vi "T1_meas_freq.vi"() -> ()   [LabVIEW 2014]
uses:
  <vilib>/Utility/file.llb/Write To Spreadsheet File (DBL).vi
  <vilib>/Utility/file.llb/Read From Spreadsheet File (DBL).vi
  <vilib>/gmath/NumericalOptimization/Nonlinear Curve Fit LM formula string.vi
  <vilib>/gmath/NI_Gmath.lvlib
  <vilib>/Analysis/NI_AALBase.lvlib
panel:
  in  "semester":string(combo)="ws17"
  out "subarray":dbl[](array[numeric])=[20.0, 40.0, 60.0, 100.0, 140.0, 180.0, 300.0, 360.0, 600.0, 800.0]
  out "appended array":dbl[](array[numeric])=[1000.0, -2000.0, 100.0]
  in  "Y-range low":dbl
  out "A":dbl[](array[numeric]) format="%.1f"
  out "T1[ms]":dbl[](array[numeric]) format="%.1f"
  out "error T1[ms]":dbl[](array[numeric]) format="%.1f"
  out "error A":dbl[](array[numeric]) format="%.1f"
  out "T1_i[ms]":dbl=100.0
  out "A_i":dbl=1000.0
  in  "Y-range high":dbl=200.0
  in  "X-range":dbl=1500.0
  out "hlim":dbl=1197.4683544303798 format="%#.1f"
  out "llim":dbl=824.4725738396625 format="%#.1f"
  out "spin echo\nsignal":dbl=7.876213904626598
  in  "time-out":u32=6
  in  "gain":u32=1000
  out "Fourier spectrum":cluster{"Y":dbl[], "Y":dbl[]}[](graph)
  in  "del T (+-)":u32=10
  in  "folder":string
  in  "don`t write data, update plot, no fit:":bool
  in  "fit:":bool
  out "XY Graph":cluster{"Y":dbl[], "Y":dbl[]}[](graph) caption="Data"
  out "error echo amplv":dbl[](array[numeric])=[0.074] format="%.3f"
  out "echo amplv":dbl[](array[numeric])=[0.745] format="%.2f"
  out "echo timev":dbl[](array[numeric])=[100.0] format="%#.1f"
  in  "many measurements:":bool=TRUE
  out "x+y":i32=2
  in  "data file":string
  out "error avg peak":dbl format="%.3f"
  out "avg peak":dbl format="%.2f"
  out "amplitude window":cluster{"Y":dbl[], "Y":dbl[]}[](graph)
  out "amplitude":cluster{"Y":dbl[], "Y":dbl[]}[](graph) caption="XY Graph"
  in  "scan freq [kHz]":u32=10
  in  "meas. time":u32=200
  in  "number meas":i32=10
  in  "spin echo time":u32=80
  in  "write data to file, update plot:":bool
  in  "single measurement:":bool=TRUE
  in  "stop":bool=TRUE
  # "peak window"
  # "1)"
  # "2)"
  # "data measured:"
  # "3)"
  # "4)"
  # "5)"
  # "fit values:"
  # "init values:"
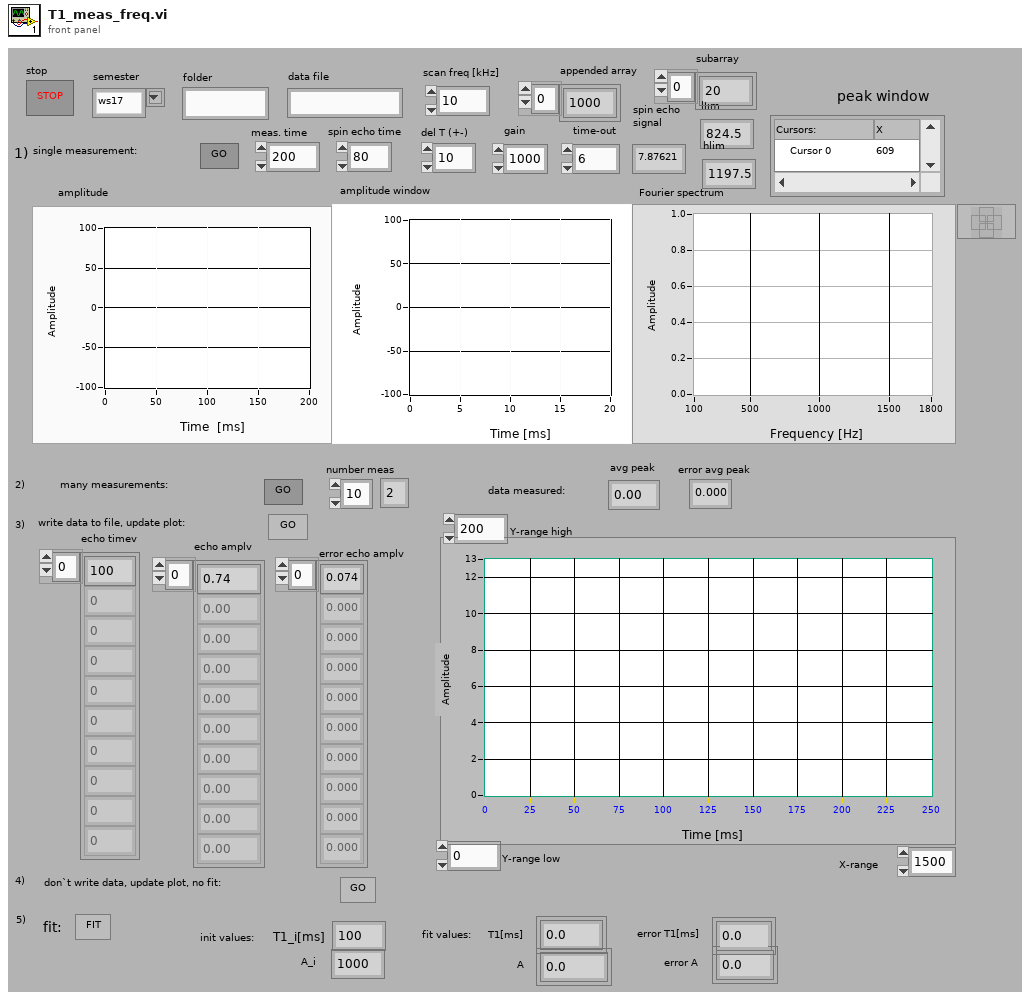
[diagram p1: front panel]
types:
  T1 = cluster{"model":string, "Parameters":string[], "x":string}
  T2 = typedef "LVCursorListTypeDef.ctl" = cluster{"Name":string, "Color":u32, "Style":u8, "Point Style":u8, "Name Visible":bool, "Allow Drag":bool, "Cursor Mode":u32, "Plot":i32, "Index":i32, "Position":cluster{"X":dbl, "Y":dbl}, "X Scale":u32, "Y Scale":u32, "Watch Plots":i32[], "Watch All Plots":bool, "Plot Area":i32, "Label Offset":cluster{"X":dbl, "Y":dbl}}[]
  T3 = typedef "NI_Matrix.lvlib/RealMatrix.ctl" = dbl[][]
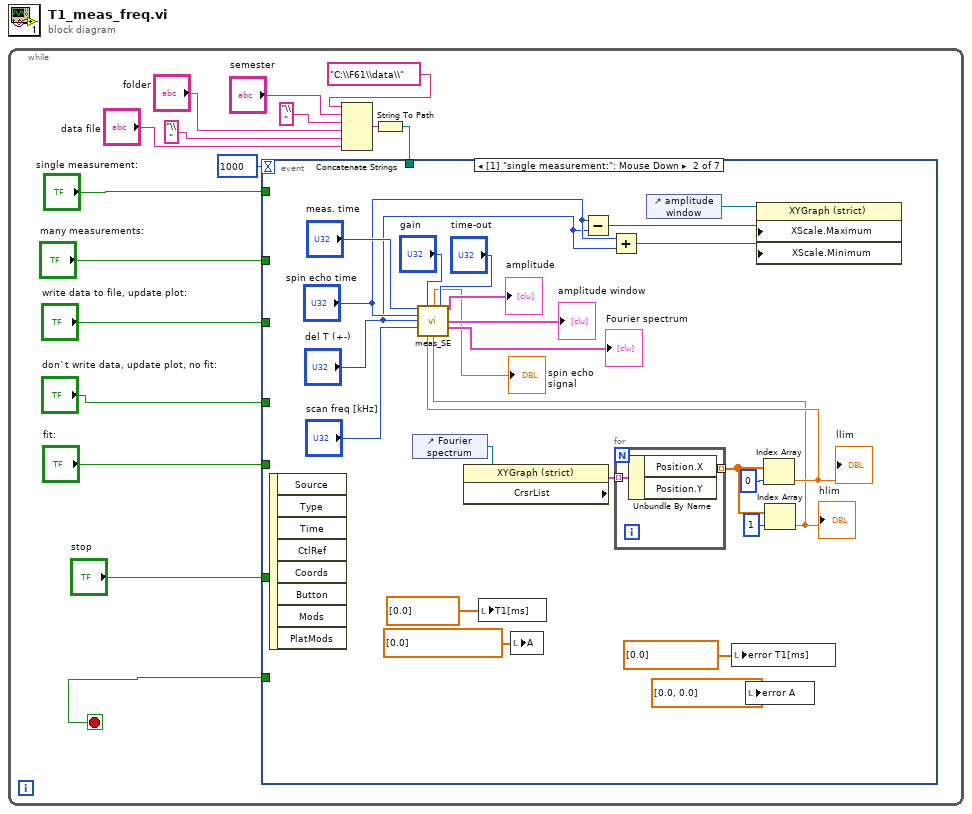
[diagram p0: block diagram]
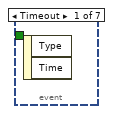
[diagram p2: hidden frame]
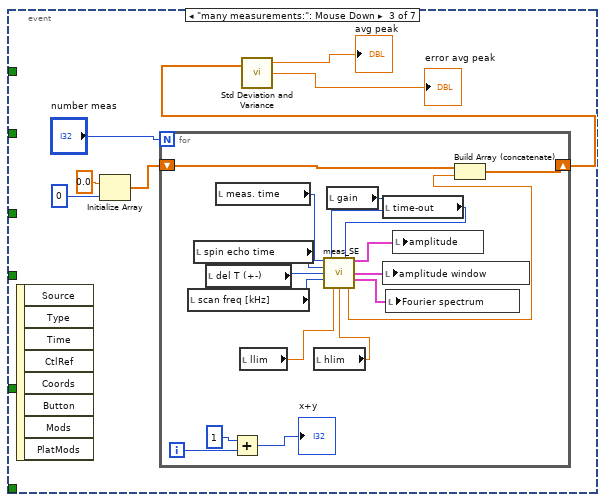
[diagram p3: hidden frame]
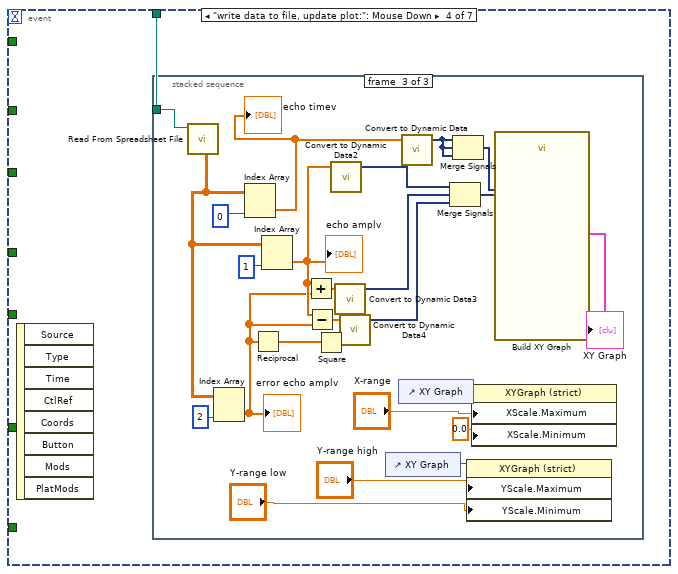
[diagram p4: hidden frame]
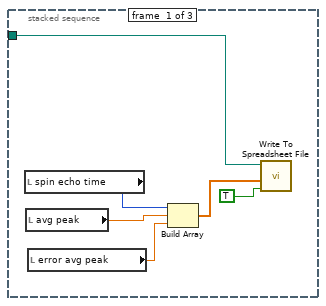
[diagram p5: hidden frame]
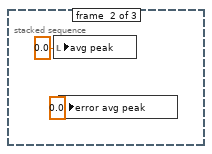
[diagram p6: hidden frame]
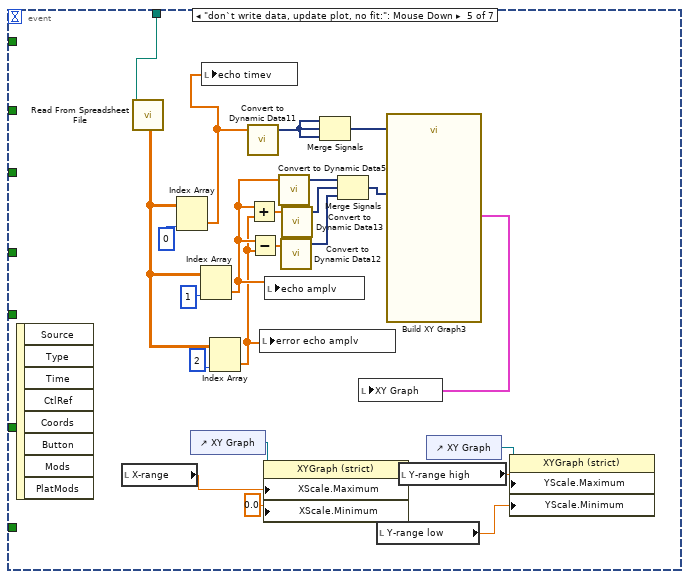
[diagram p7: hidden frame]
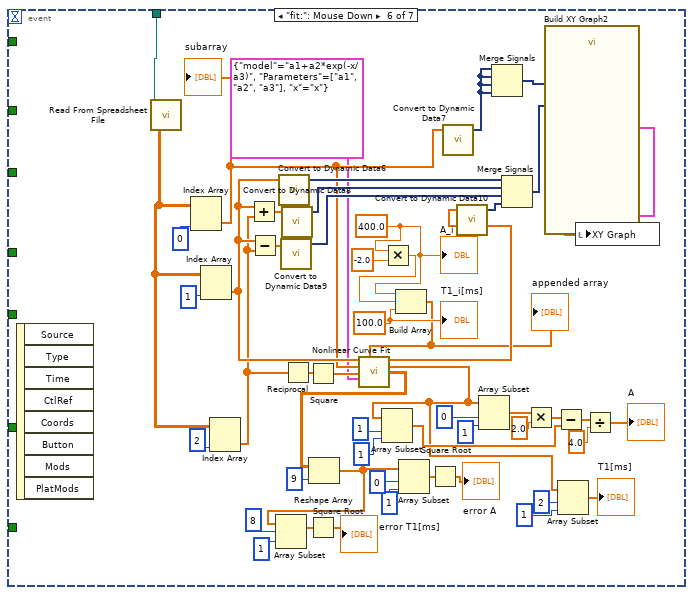
[diagram p8: hidden frame]
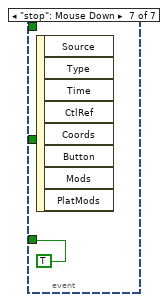
[diagram p9: hidden frame]
diagram:
  n1 = while {
    stop <- w9 stop-if-true
    n2 = Concatenate Strings("C:\\F61\\data\\", "semester", "\\" ("string"), "folder", "\\" ("string"), "data file") -> (w14:string)
    n3 = String To Path(string=w14) -> (path=w13:path)
    n4 = event shown="[1] \"single measurement:\": Mouse Down" {
      selector: _ -> [_ _ _ _ _ _ _]
      dyn-events: _ -> [_ _ _ _ _ _ _]
      timeout: 1000 -> [_ _ _ _ _ _ _]
      tunnel: "single measurement:" -> [_ _ _ _ _ _ _]
      tunnel: "write data to file, update plot:" -> [_ _ _ _ _ _ _]
      tunnel: w13 -> [_ _ _ w67 w111 w157 _]
      tunnel: "many measurements:" -> [_ _ _ _ _ _ _]
      tunnel: "fit:" -> [_ _ _ _ _ _ _]
      tunnel: "stop" -> [_ _ _ _ _ _ _]
      tunnel: [_ _ _ _ _ _ TRUE ("stop")] -> w9
      tunnel: "don`t write data, update plot, no fit:" -> [_ _ _ _ _ _ _]
      event Timeout {
        n5 = event-data() -> ()  [unwired: 1 in, 2 out]
      }
      event "single measurement:": Mouse Down {
        n6 = event-data() -> ()  [unwired: 1 in, 8 out]
        n7 = control-ref of="Fourier spectrum"() -> (w40:refnum<vi>)
        n8 = property class="XYGraph (strict)"(reference=w40) -> ("CrsrList"=w39:T2)  [unwired: 1 in, 2 out]
        n9 = local write "T1[ms]"(dbl[] [0.0] ("T1[ms]")) -> ()
        n10 = local write "A"(dbl[] [0.0] ("A")) -> ()
        n11 = Subtract(x="spin echo time", y="del T (+-)") -> (x-y=w23:u32)
        n12 = Add(x="spin echo time", y="del T (+-)") -> (x+y=w22:u32)
        n13 = for {
          tunnel: w39 -> [w42] mode=indexing
          tunnel: [w41] -> w38 mode=indexing
          n14 = Unbundle By Name(w42) -> ("Position.X"=w41:dbl)  [unwired: 1 out]
        }
        n15 = control-ref of="amplitude window"() -> (w26:refnum<vi>)
        n16 = local write "error T1[ms]"(dbl[] [0.0] ("error T1[ms]")) -> ()
        n17 = local write "error A"(dbl[] [0.0, 0.0] ("error A")) -> ()
        n18 = property class="XYGraph (strict)"(reference=w26, "XScale.Maximum"=w23, "XScale.Minimum"=w22) -> ()  [unwired: 1 in, 2 out]
        n19 = Index Array(array=w38, index=0) -> (element=w28:dbl)
        "llim" <- w28
        n20 = Index Array(array=w38, index=1) -> (element=w27:dbl)
        "hlim" <- w27
        n21 = call "meas_SE.vi"("meas. time [ms]"="meas. time", "gainfac"="gain", "time out [s]"="time-out", "spin echo time [ms]"="spin echo time", "del T (+-) ][ms]"="del T (+-)", "scan freq [kHz]"="scan freq [kHz]", "llim"=w28, "hlim"=w27) -> ("SE"=→"spin echo\nsignal":dbl, "Amplitude"=→"amplitude":cluster{"Y":dbl[], "Y":dbl[]}[], "Spin echo (time)"=→"amplitude window":cluster{"Y":dbl[], "Y":dbl[]}[], "Spin echo (freq)"=→"Fourier spectrum":cluster{"Y":dbl[], "Y":dbl[]}[])  [unwired: 3 in, 1 out]
      }
      event "many measurements:": Mouse Down {
        n22 = event-data() -> ()  [unwired: 1 in, 8 out]
        n23 = Initialize Array(0.0 ("element"), 0 ("dimension size")) -> (w47:dbl[])
        n24 = for {
          N: "number meas" -> [_]
          shift-right: [w62] -> w46
          shift-left: w47 -> [w63]
          i -> [w65]
          n25 = local read "scan freq [kHz]"() -> (w58:u32)
          n26 = local read "spin echo time"() -> (w60:u32)
          n27 = local read "del T (+-)"() -> (w59:u32)
          n28 = local read "meas. time"() -> (w61:u32)
          n29 = Add(x=1, y=w65) -> (x+y=→"x+y":i32)
          n30 = local read "llim"() -> (w54:dbl)
          n31 = local read "hlim"() -> (w53:dbl)
          n32 = local read "gain"() -> (w57:u32)
          n33 = local read "time-out"() -> (w56:u32)
          n34 = call "meas_SE.vi"("meas. time [ms]"=w61, "gainfac"=w57, "time out [s]"=w56, "spin echo time [ms]"=w60, "del T (+-) ][ms]"=w59, "scan freq [kHz]"=w58, "llim"=w54, "hlim"=w53) -> ("Amplitude"=w52:cluster{"Y":dbl[], "Y":dbl[]}[], "Spin echo (time)"=w51:cluster{"Y":dbl[], "Y":dbl[]}[], "Spin echo (freq)"=w50:cluster{"Y":dbl[], "Y":dbl[]}[], "SE-corr"=w55:dbl)  [unwired: 3 in, 1 out]
          n35 = local write "amplitude window"(w51) -> ()
          n36 = local write "Fourier spectrum"(w50) -> ()
          n37 = local write "amplitude"(w52) -> ()
          n38 = Build Array (concatenate)(w63, w55) -> (w62:dbl[])
        }
        n39 = call <vilib>:"Std Deviation and Variance.vi"("X"=w46) -> ("mean"=→"avg peak":dbl, "standard deviation"=→"error avg peak":dbl)  [unwired: 1 in, 1 out]
      }
      event "write data to file, update plot:": Mouse Down {
        n40 = event-data() -> ()  [unwired: 1 in, 8 out]
        n41 = stacked-sequence {
          tunnel: w67 -> [w68 _ w99]
          frame #0 {
            n42 = local read "spin echo time"() -> (w69:u32)
            n43 = local read "avg peak"() -> (w70:dbl)
            n44 = local read "error avg peak"() -> (w73:dbl)
            n45 = Build Array(w69, w70, w73) -> (w71:dbl[])
            n46 = call-poly <vilib>:"Write To Spreadsheet File.vi"("append to file? (new file:F)"=TRUE, "1D data"=w71, "file path (dialog if empty)"=w68) -> ()  [unwired: 5 in, 1 out]
          }
          frame #1 {
            n47 = local write "avg peak"(sgl 0.0 ("avg diff")) -> ()
            n48 = local write "error avg peak"(0.0 ("error avg diff")) -> ()
          }
          frame #2 {
            n49 = call-poly <vilib>:"Read From Spreadsheet File.vi"("file path (dialog if empty)"=w99) -> ("all rows"=w98:dbl[][])  [unwired: 6 in, 4 out]
            n50 = Index Array(array=w98, index (col)=2 ("index (row)")) -> (element=w84:dbl[])  [unwired: 1 in]
            "error echo amplv" <- w84
            n51 = Index Array(array=w98, index (col)=0 ("index (row)")) -> (element=w82:dbl[])  [unwired: 1 in]
            "echo timev" <- w82
            n52 = Reciprocal(x=w84) -> (1/x=w83:dbl[])
            n53 = Index Array(array=w98, index (col)=1 ("index (row)")) -> (element=w85:dbl[])  [unwired: 1 in]
            "echo amplv" <- w85
            n54 = Add(x=w85, y=w84) -> (x+y=w89:dbl[])
            n55 = Subtract(x=w85, y=w84) -> (x-y=w88:dbl[])
            n56 = Square(x=w83) -> ()  [unwired: 1 out]
            n57 = call "Convert to Dynamic Data2"("Array"=w85) -> ("Dynamic Data Type"=w90:dynamicdata)  [unwired: 3 in]
            n58 = call "Convert to Dynamic Data3"("Array"=w89) -> ("Dynamic Data Type"=w87:dynamicdata)  [unwired: 3 in]
            n59 = call "Convert to Dynamic Data4"("Array"=w88) -> ("Dynamic Data Type"=w86:dynamicdata)  [unwired: 3 in]
            n60 = control-ref of="XY Graph"() -> (w78:refnum<vi>)
            n61 = control-ref of="XY Graph"() -> (w81:refnum<vi>)
            n62 = call "Convert to Dynamic Data"("Array"=w82) -> ("Dynamic Data Type"=w93:dynamicdata)  [unwired: 3 in]
            n63 = Merge Signals(w90, w87, w86) -> (w91:dynamicdata)
            n64 = Merge Signals(w93, w93, w93) -> (w92:dynamicdata)
            n65 = property class="XYGraph (strict)"(reference=w78, "YScale.Maximum"="Y-range high", "YScale.Minimum"="Y-range low") -> ()  [unwired: 1 in, 2 out]
            n66 = property class="XYGraph (strict)"(reference=w81, "XScale.Maximum"="X-range", "XScale.Minimum"=0.0 ("X Scale.Range:Maximum")) -> ()  [unwired: 1 in, 2 out]
            n67 = call "Build XY Graph"("Y Input"=w91, "X Input"=w92) -> ("XY Graph"=→"XY Graph":cluster{"Y":dbl[], "Y":dbl[]}[])  [unwired: 8 in, 1 out]
          }
        }
      }
      event "don`t write data, update plot, no fit:": Mouse Down {
        n68 = event-data() -> ()  [unwired: 1 in, 8 out]
        n69 = local read "X-range"() -> (w104:dbl)
        n70 = call-poly <vilib>:"Read From Spreadsheet File.vi"("file path (dialog if empty)"=w111) -> ("all rows"=w122:dbl[][])  [unwired: 6 in, 4 out]
        n71 = Index Array(array=w122, index (col)=0 ("index (row)")) -> (element=w108:dbl[])  [unwired: 1 in]
        n72 = control-ref of="XY Graph"() -> (w103:refnum<vi>)
        n73 = Index Array(array=w122, index (col)=1 ("index (row)")) -> (element=w107:dbl[])  [unwired: 1 in]
        n74 = local write "echo timev"(w108) -> ()
        n75 = Index Array(array=w122, index (col)=2 ("index (row)")) -> (element=w106:dbl[])  [unwired: 1 in]
        n76 = call "Convert to Dynamic Data11"("Array"=w108) -> ("Dynamic Data Type"=w109:dynamicdata)  [unwired: 3 in]
        n77 = Add(x=w107, y=w106) -> (x+y=w115:dbl[])
        n78 = Subtract(x=w107, y=w106) -> (x-y=w114:dbl[])
        n79 = local write "error echo amplv"(w106) -> ()
        n80 = property class="XYGraph (strict)"(reference=w103, "XScale.Maximum"=w104, "XScale.Minimum"=0.0 ("X Scale.Range:Maximum")) -> ()  [unwired: 1 in, 2 out]
        n81 = local write "echo amplv"(w107) -> ()
        n82 = call "Convert to Dynamic Data5"("Array"=w107) -> ("Dynamic Data Type"=w116:dynamicdata)  [unwired: 3 in]
        n83 = call "Convert to Dynamic Data12"("Array"=w114) -> ("Dynamic Data Type"=w112:dynamicdata)  [unwired: 3 in]
        n84 = call "Convert to Dynamic Data13"("Array"=w115) -> ("Dynamic Data Type"=w113:dynamicdata)  [unwired: 3 in]
        n85 = Merge Signals(w109, w109, w109) -> (w118:dynamicdata)
        n86 = Merge Signals(w116, w113, w112) -> (w117:dynamicdata)
        n87 = local read "Y-range low"() -> (w100:dbl)
        n88 = call "Build XY Graph3"("Y Input"=w117, "X Input"=w118) -> ("XY Graph"=w110:cluster{"Y":dbl[], "Y":dbl[]}[])  [unwired: 8 in, 1 out]
        n89 = local write "XY Graph"(w110) -> ()
        n90 = local read "Y-range high"() -> (w101:dbl)
        n91 = control-ref of="XY Graph"() -> (w102:refnum<vi>)
        n92 = property class="XYGraph (strict)"(reference=w102, "YScale.Maximum"=w101, "YScale.Minimum"=w100) -> ()  [unwired: 1 in, 2 out]
      }
      event "fit:": Mouse Down {
        w150 = 100.0 ("element")
        w152 = 400.0 ("A")
        n93 = event-data() -> ()  [unwired: 1 in, 8 out]
        n94 = call-poly <vilib>:"Read From Spreadsheet File.vi"("file path (dialog if empty)"=w157) -> ("all rows"=w175:dbl[][])  [unwired: 6 in, 4 out]
        n95 = Index Array(array=w175, index (col)=0 ("index (row)")) -> (element=w158:dbl[])  [unwired: 1 in]
        "subarray" <- w158
        n96 = Index Array(array=w175, index (col)=1 ("index (row)")) -> (element=w164:dbl[])  [unwired: 1 in]
        n97 = Index Array(array=w175, index (col)=2 ("index (row)")) -> (element=w163:dbl[])  [unwired: 1 in]
        n98 = Add(x=w164, y=w163) -> (x+y=w168:dbl[])
        n99 = Subtract(x=w164, y=w163) -> (x-y=w167:dbl[])
        n100 = call "Convert to Dynamic Data6"("Array"=w164) -> ("Dynamic Data Type"=w169:dynamicdata)  [unwired: 3 in]
        n101 = call "Convert to Dynamic Data9"("Array"=w167) -> ("Dynamic Data Type"=w165:dynamicdata)  [unwired: 3 in]
        n102 = call "Convert to Dynamic Data8"("Array"=w168) -> ("Dynamic Data Type"=w166:dynamicdata)  [unwired: 3 in]
        n103 = Reciprocal(x=w163) -> (1/x=w162:dbl[])
        n104 = Square(x=w162) -> (x^2=w161:dbl[])
        n105 = Multiply(x=w152, y=-2.0) -> (x*y=w151:dbl)
        n106 = Build Array(w152, w151, w150) -> (w149:dbl[])
        "appended array" <- w149
        n107 = call-poly <vilib>:"Nonlinear Curve Fit.vi"("Y"=w164, "initial parameters"=w149, "X"=w158, "Weight"=w161, "model description"=T1 {"model"="a1+a2*exp(-x/a3)", "Parameters"=["a1", "a2", "a3"], "x"="x"}) -> ("best nonlinear fit"=w160:dbl[], "best fit parameters"=w123:dbl[], "covariance"=w124:T3)  [unwired: 6 in, 2 out]
        n108 = Reshape Array(w124, 9 ("index")) -> (w139:dbl[])
        n109 = Array Subset(array=w139, index=8, length=1 ("index")) -> (w136:dbl[])
        n110 = Square Root(x=w136) -> (sqrt(x)=→"error T1[ms]":dbl[])
        n111 = Array Subset(array=w123, index=1, length=1) -> (w128:dbl[])
        n112 = Array Subset(array=w139, index=0, length=1) -> (w141:dbl[])
        n113 = Square Root(x=w141) -> (sqrt(x)=→"error A":dbl[])
        n114 = call "Convert to Dynamic Data7"("Array"=w158) -> ("Dynamic Data Type"=w154:dynamicdata)  [unwired: 3 in]
        n115 = call "Convert to Dynamic Data10"("Array"=w160) -> ("Dynamic Data Type"=w159:dynamicdata)  [unwired: 3 in]
        n116 = Array Subset(array=w123, index=0, length=1) -> (w130:dbl[])
        n117 = Merge Signals(w154, w154, w154, w154) -> (w171:dynamicdata)
        n118 = Merge Signals(w169, w166, w165, w159) -> (w170:dynamicdata)
        n119 = Multiply(x=w130, y=2.0) -> (x*y=w129:dbl[])
        n120 = call "Build XY Graph2"("Y Input"=w170, "X Input"=w171) -> ("XY Graph"=w155:cluster{"Y":dbl[], "Y":dbl[]}[])  [unwired: 8 in, 1 out]
        n121 = Subtract(x=w129, y=w128) -> (x-y=w127:dbl[])
        n122 = Array Subset(array=w123, index=2, length=1) -> (→"T1[ms]":dbl[])
        n123 = local write "XY Graph"(w155) -> ()
        n124 = Divide(x=w127, y=4.0) -> (x/y=→"A":dbl[])
        "A_i" <- w152
        "T1_i[ms]" <- w150
      }
      event "stop": Mouse Down {
        n125 = event-data() -> ()  [unwired: 1 in, 8 out]
      }
    }
  }
